vi "ReadDataFile_V1.vi"(8 "error in (no error)":errorcluster, 9 "Create CSV files?":bool, 10 "Channel Names Array":string[](array[string]), 11 "DataFolder Path":path) -> (0 "error out":errorcluster, 2 "Current Measurements":cluster{dbl[], dbl[]}[](array[cluster]), 3 "Voltage Measurements":cluster{dbl[], dbl[]}[](array[cluster]))   [LabVIEW 2019]
uses:
  <vilib>/Utility/file.llb/Write Delimited Spreadsheet (string).vi
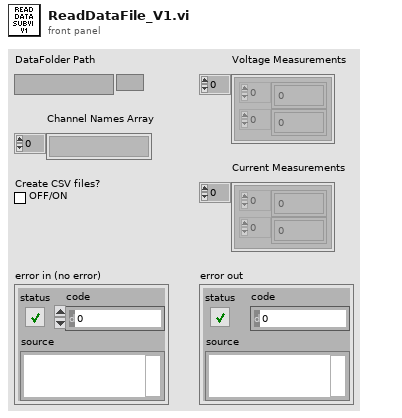
[diagram p1: front panel]
types:
  T1 = enum16{"big-endian, network order", "native, host order", "little-endian"}
  T2 = cluster{"Array of fetched data":dbl[][], string, i32[]}
  T3 = enum16{"open", "replace", "create", "open or create", "replace or create", "replace or create with confirmation"}
  T4 = cluster{"Array of fetched data":dbl[][], string, i32[]}[]
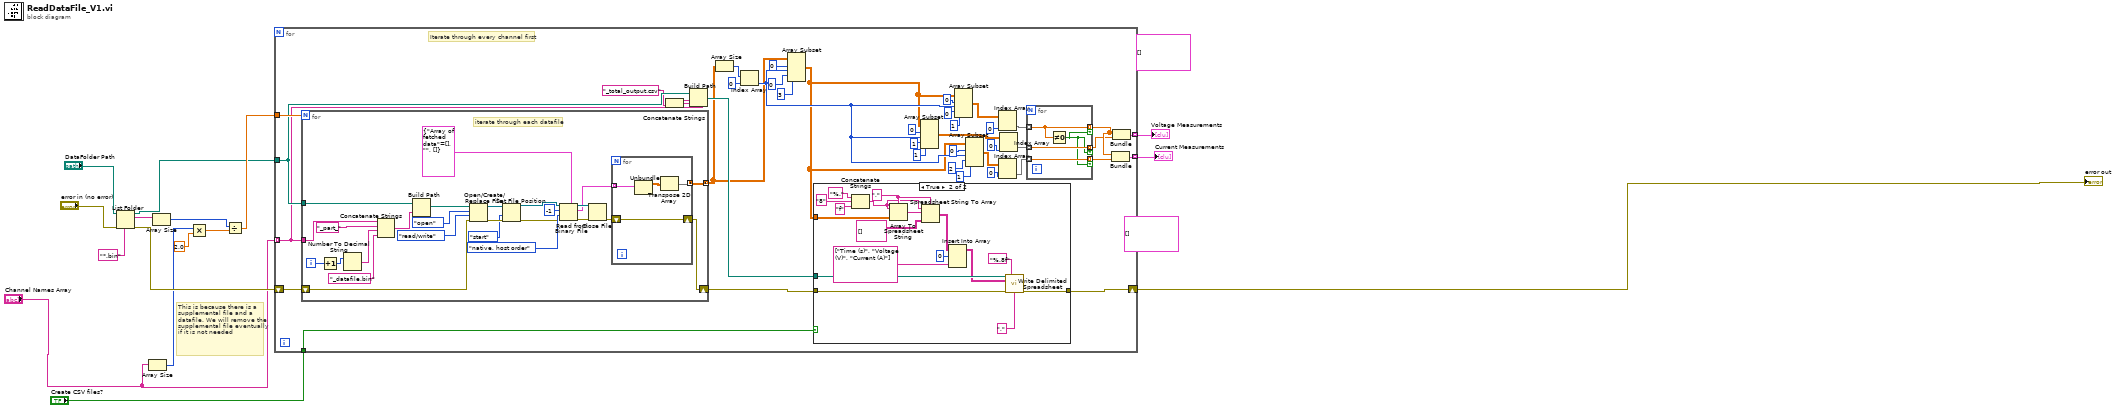
[diagram p0: block diagram]
diagram:
  (unwired) cluster{dbl[], dbl[]}[] []
  (unwired) cluster{dbl[], dbl[]}[] []
  # "This is because there is a supplemental file and a datafile. We will remove the supplemental file eventually if it is not needed"
  n1 = List Folder(path="DataFolder Path", pattern="*.bin", error in="error in (no error)") -> (path out=w9:path, filenames=w4:string[], error out=w11:errorcluster)  [unwired: 1 in, 1 out]
  n2 = Array Size(array="Channel Names Array") -> (size(s)=w8:i32)
  n3 = Array Size(array=w4) -> (size(s)=w7:i32)
  n4 = Multiply(x=w8, y=2.0) -> (x*y=w6:dbl)
  n5 = Divide(x=w7, y=w6) -> (x/y=w10:dbl)
  n6 = for {
    tunnel: w9 -> [w53]
    tunnel: "Channel Names Array" -> [w51] mode=indexing
    tunnel: w10 -> [w57]
    shift-right: [w47] -> w1
    shift-left: w11 -> [w56]
    tunnel: [w33] -> w12 mode=indexing
    tunnel: [w32] -> w13 mode=indexing
    tunnel: "Create CSV files?" -> [w19]
    # "Iterate through every channel first"
    n7 = for {
      N: w57 -> [_]
      tunnel: w51 -> [w105]
      tunnel: w53 -> [w101]
      shift-right: [w81] -> w48
      shift-left: w56 -> [w96]
      tunnel: [w80] -> w18 mode=concatenating
      i -> [w85]
      # "iterate through each datafile"
      n8 = Increment(x=w85) -> (x+1=w84:i32)
      n9 = Number To Decimal String(number=w84) -> (decimal integer string=w103:string)  [unwired: 1 in]
      n10 = Concatenate Strings(w105, "_part_" ("string"), w103, "_datafile.bin" ("string")) -> (w100:string)
      n11 = Build Path(base path=w101, name or relative path=w100) -> (appended path=w99:path)
      n12 = Open/Create/Replace File(file path (use dialog)=w99, error in=w96, operation (0:open)=T3."open", access (0:read/write)=enum16{"read/write", "read-only", "write-only"}."read/write") -> (refnum out=w89:refnum<file>, error out=w90:errorcluster)  [unwired: 2 in, 1 out]
      n13 = Set File Position(refnum=w89, from (0:start)=enum16{"start", "end", "current"}."start", error in=w90) -> (refnum out=w86:refnum<file>, error out=w87:errorcluster)  [unwired: 1 in]
      n14 = Read from Binary File(5:T2 {"Array of fetched data"=[], "", []} ("cluster"), 8:w87, 9:T1."native, host order" ("byte order (0:big-endian, network order)"), 10:-1 ("count (1)"), 11:w86) -> (0:w92:errorcluster, 2:w83:T4, 3:w91:refnum<file>)  [unwired: 1 in, 1 out]
      n15 = Close File(refnum=w91, error in=w92) -> (error out=w82:errorcluster)  [unwired: 1 out]
      n16 = for {
        tunnel: w83 -> [w109] mode=indexing
        tunnel: [w106] -> w80 mode=concatenating
        shift-right: [w108] -> w81
        shift-left: w82 -> [w108]
        n17 = Unbundle(w109) -> ("Array of fetched data"=w107:dbl[][])  [unwired: 2 out]
        n18 = Transpose 2D Array(2D array=w107) -> (transposed array=w106:dbl[][])
      }
    }
    n19 = Concatenate Strings(w51, "_total_output.csv" ("string")) -> (w52:string)
    n20 = Build Path(base path=w53, name or relative path=w52) -> (appended path=w49:path)
    n21 = Array Size(array=w18) -> (size(s)=w55:i32[])
    n22 = Index Array(array=w55, index=0) -> (element=w34:i32)
    n23 = Array Subset(array=w18, index (row)=0 ("index"), length (row)=w34, index (col)=0 ("index"), length (col)=3 ("length")) -> (w17:dbl[][])
    n24 = case shown="True" w19 {
      tunnel: w49 -> [_ w75]
      tunnel: w48 -> [w58 w74]
      tunnel: [w58 w73] -> w47
      tunnel: w17 -> [_ w65]
      frame False {
      }
      frame True {
        w70 = "," ("delimiter (Tab)")
        n25 = Concatenate Strings("%." ("string"), "8" ("string"), "f" ("string")) -> (w66:string)
        n26 = Array To Spreadsheet String(delimiter (Tab)=w70, array=w65, 3:w66) -> (spreadsheet string=w69:string)
        n27 = Spreadsheet String To Array(delimiter (Tab)=w70, format string=w66, spreadsheet string=w69, array type (2D Dbl)=string[][] []) -> (array=w63:string[][])
        n28 = Insert Into Array(array=w63, index (row)=0, new element=string[] ["Time (s)", "Voltage (V)", "Current (A)"]) -> (w61:string[][])  [unwired: 1 in]
        n29 = call-poly <vilib>:"Write Delimited Spreadsheet.vi"("file path (dialog if empty)"=w75, "format (%s)"="%.8f" ("format (%.3f)"), "2D data"=w61, "error in (no error)"=w74, "delimiter (\\t)"="," ("delimiter (\\t)")) -> ("error out"=w73:errorcluster)  [unwired: 9 in, 1 out]
      }
    }
    n30 = Array Subset(array=w17, index (row)=0 ("index"), length (row)=w34, index (col)=1 ("index"), length (col)=1 ("length")) -> (w30:dbl[][])
    n31 = Array Subset(array=w17, index (row)=0 ("index"), length (row)=w34, index (col)=0 ("index"), length (col)=1 ("length")) -> (w31:dbl[][])
    n32 = Array Subset(array=w17, index (row)=0 ("index"), length (row)=w34, index (col)=2 ("index"), length (col)=1 ("length")) -> (w29:dbl[][])
    n33 = Index Array(array=w31, index (col)=0 ("disabled index (col)")) -> (element=w25:dbl[])  [unwired: 1 in]
    n34 = Index Array(array=w29, index (col)=0 ("disabled index (col)")) -> (element=w23:dbl[])  [unwired: 1 in]
    n35 = Index Array(array=w30, index (col)=0 ("disabled index (col)")) -> (element=w24:dbl[])  [unwired: 1 in]
    n36 = for {
      tunnel: w25 -> [w76] mode=indexing
      tunnel: w24 -> [w79] mode=indexing
      tunnel: w23 -> [w78] mode=indexing
      tunnel: [w76] -> w22 mode=indexing if=w77
      tunnel: [w79] -> w21 mode=indexing if=w77
      tunnel: [w78] -> w20 mode=indexing if=w77
      n37 = Not Equal To 0?(x=w76) -> (x != 0?=w77:bool)
    }
    n38 = Bundle(w22, w20) -> (w32:cluster{dbl[], dbl[]})  [unwired: 1 in]
    n39 = Bundle(w22, w21) -> (w33:cluster{dbl[], dbl[]})  [unwired: 1 in]
  }
  "Current Measurements" <- w13
  "Voltage Measurements" <- w12
  "error out" <- w1
